vi "Get Dashboard Data.vi"   [LabVIEW 2012]
uses:
  BotStatus.vi
types:
  T1 = cluster{"Target Position X":dbl, "Target Position Y":dbl, "Target Found":bool}
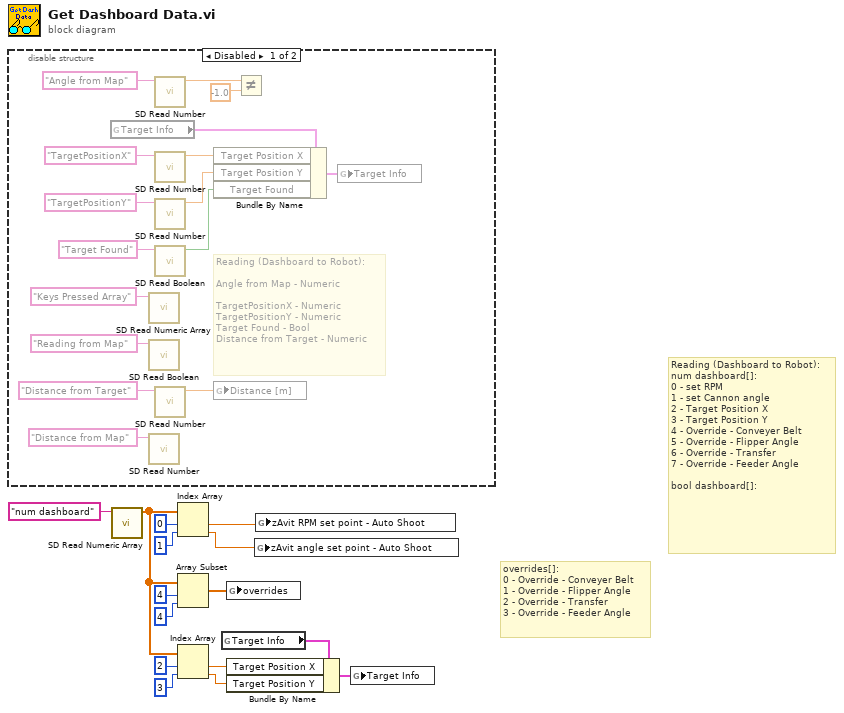
[diagram p0: block diagram]
diagram:
  # "overrides[]:\n0 - Override - Conveyer Belt\n1 - Override - Flipper Angle \n2 - Override - Transfer\n3 - Override - Feeder Angle"
  # "Reading (Dashboard to Robot):\nnum dashboard[]:\n0 - set RPM\n1 - set Cannon angle\n2 - Target Position X\n3 - Target Position Y\n4 - Override - Conveyer Belt\n5 - Override - Flipper Angle \n6 - Override - Transfer\n7 - Override - Feeder Angle\n\nbool dashboard[]:"
  n1 = disable-structure shown="Disabled" {
    frame Disabled {
      # "Reading (Dashboard to Robot):\n\nAngle from Map - Numeric\n\nTargetPositionX - Numeric\nTargetPositionY - Numeric\nTarget Found - Bool\nDistance from Target - Numeric"
      n2 = global read "BotStatus.vi" "Target Info"() -> (w20:T1)
      n3 = call <vilib>:"SD Read Numeric Array.vi"("Name"="Keys Pressed Array") -> ()  [unwired: 8 in, 3 out]
      n4 = call <vilib>:"SD Read Boolean.vi"("Name"="Reading from Map") -> ()  [unwired: 8 in, 3 out]
      n5 = call <vilib>:"SD Read Number.vi"("Name"="Distance from Map") -> ()  [unwired: 8 in, 3 out]
      n6 = call <vilib>:"SD Read Number.vi"("Name"="Angle from Map") -> ("Numeric"=w27:dbl)  [unwired: 8 in, 2 out]
      n7 = call <vilib>:"SD Read Number.vi"("Name"="TargetPositionX") -> ("Numeric"=w21:dbl)  [unwired: 8 in, 2 out]
      n8 = call <vilib>:"SD Read Number.vi"("Name"="TargetPositionY") -> ("Numeric"=w22:dbl)  [unwired: 8 in, 2 out]
      n9 = call <vilib>:"SD Read Boolean.vi"("Name"="Target Found") -> ("Boolean"=w23:bool)  [unwired: 8 in, 2 out]
      n10 = call <vilib>:"SD Read Number.vi"("Name"="Distance from Target") -> ("Numeric"=w25:dbl)  [unwired: 8 in, 2 out]
      n11 = Bundle By Name(cluster=w20, "Target Position X"=w21, "Target Position Y"=w22, "Target Found"=w23) -> (w24:T1)
      n12 = global write "BotStatus.vi" "Distance [m]"(w25) -> ()
      n13 = Not Equal?(x=w27, y=-1.0) -> ()  [unwired: 1 out]
      n14 = global write "BotStatus.vi" "Target Info"(w24) -> ()
    }
    frame Enabled {
    }
  }
  n15 = call <vilib>:"SD Read Numeric Array.vi"("Name"="num dashboard") -> ("Numeric Array"=w4:dbl[])  [unwired: 8 in, 2 out]
  n16 = Index Array(array=w4, index #1=0 ("index"), index #2=1 ("index")) -> (element #1=w2:dbl, element #2=w1:dbl)
  n17 = Array Subset(array=w4, index=4, length=4) -> (w12:dbl[])
  n18 = Index Array(array=w4, index #1=2 ("index"), index #2=3 ("index")) -> (element #1=w8:dbl, element #2=w7:dbl)
  n19 = global read "BotStatus.vi" "Target Info"() -> (w11:T1)
  n20 = global write "BotStatus.vi" "overrides"(w12) -> ()
  n21 = Bundle By Name(cluster=w11, "Target Position X"=w8, "Target Position Y"=w7) -> (w3:T1)
  n22 = global write "BotStatus.vi" "zAvit angle set point - Auto Shoot"(w1) -> ()
  n23 = global write "BotStatus.vi" "zAvit RPM set point - Auto Shoot"(w2) -> ()
  n24 = global write "BotStatus.vi" "Target Info"(w3) -> ()
